vi "Practica 6.vi"() -> ()   [LabVIEW 2018]
uses:
  <vilib>/LabVIEW Interface for Arduino/Type Defs/Digital Pin.ctl
  <vilib>/LabVIEW Interface for Arduino/Type Defs/Pin Mode.ctl
  <vilib>/LabVIEW Interface for Arduino/LabVIEW Interface for Arduino.lvlib
  <vilib>/ptbypt/NI_PtbyPt.lvlib
panel:
  in  "stop":bool
  out "Contador":dbl
  out "Impulso":bool
  in  "Seleccion de PIN":T1
  # "Practica 6:Contador de Impulsos \nen una Entrada Digital"
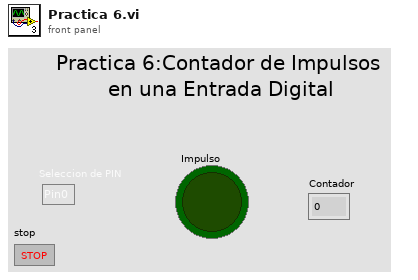
[diagram p1: front panel]
types:
  T1 = typedef "LabVIEW Interface for Arduino.lvlib/Digital Pin.ctl" = enum8{"Pin0", "Pin1", "Pin2", "Pin3", "Pin4", "Pin5", "Pin6", "Pin7", "Pin8", "Pin9", "Pin10", "Pin11", "Pin12", "Pin13"}
  T2 = typedef "LabVIEW Interface for Arduino.lvlib/Arduino Resource.ctl" = cluster{"VISA resource":refnum<visa-resource-name>, "Board Type":T3, "Connection Type":enum8{"USB / Serial"}, "Bytes Per Packet (15)":u8}
  T3 = typedef "LabVIEW Interface for Arduino.lvlib/Board Type.ctl" = enum16{"Uno", "Dimuelanove w/Atmega 328", "Mega 2560"}
  T4 = typedef "LabVIEW Interface for Arduino.lvlib/Pin Mode.ctl" = enum8{"Input", "Output"}
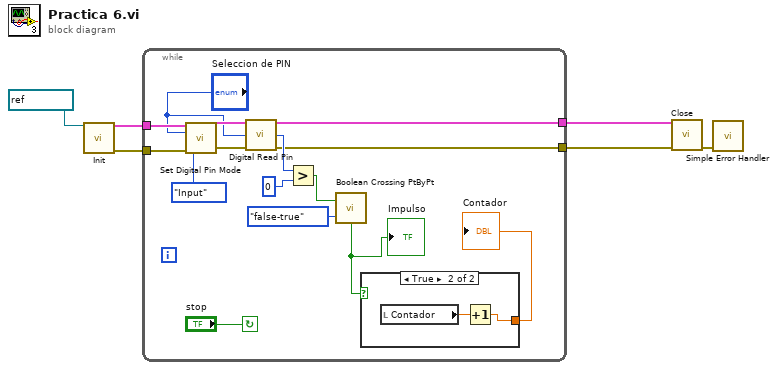
[diagram p0: block diagram]
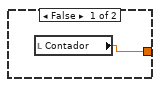
[diagram p2: hidden frame]
diagram:
  n1 = call <vilib>:"Init.vi"("VISA resource"=refnum<visa-resource-name> "COM9") -> ("Arduino Resource"=w5:T2, "error out"=w4:errorcluster)  [unwired: 17 in]
  n2 = while {
    tunnel: w5 -> [w20]
    tunnel: w4 -> [w19]
    tunnel: [w10] -> w2
    tunnel: [w9] -> w1
    stop <- "stop" continue-if-true
    n3 = call <vilib>:"Set Digital Pin Mode.vi"("Arduino Resource"=w20, "Digital I/O Pin"="Seleccion de PIN", "Pin Mode (Input)"=Pin_Mode."Input", "error in"=w19) -> ("Arduino Resource"=w17:T2, "error out"=w18:errorcluster)  [unwired: 10 in]
    n4 = call <vilib>:"Digital Read Pin.vi"("Arduino Resource"=w17, "Digital I/O Pin (0)"="Seleccion de PIN", "error in"=w18) -> ("Arduino Resource"=w9:T2, "Value"=w14:u8, "error out"=w10:errorcluster)  [unwired: 10 in]
    n5 = Greater?(x=w14, y=0) -> (0:w12:bool)
    n6 = call <vilib>:"Boolean Crossing PtByPt.vi"("direction"=enum16{"either", "false-true", "true-false"}."false-true", "input"=w12) -> ("crossing"=w8:bool)  [unwired: 1 in]
    "Impulso" <- w8
    n7 = case shown="True" w8 {
      tunnel: [w22 w24] -> w7
      frame False {
        n8 = local read "Contador"() -> (w22:dbl)
      }
      frame True {
        n9 = local read "Contador"() -> (w23:dbl)
        n10 = Increment(x=w23) -> (x+1=w24:dbl)
      }
    }
    "Contador" <- w7
  }
  n11 = call <vilib>:"Close.vi"("Arduino Resource"=w1, "error in"=w2) -> ("error out"=w3:errorcluster)  [unwired: 13 in]
  n12 = call <vilib>:"Simple Error Handler.vi"("error in (no error)"=w3) -> ()  [unwired: 4 in, 5 out]
